vi "例4-20.vi"   [LabVIEW 2019]
uses:
  <vilib>/Utility/file.llb/Write Delimited Spreadsheet (DBL).vi
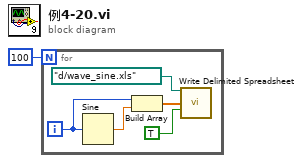
[diagram p0: block diagram]
diagram:
  n1 = for {
    N: 100 -> [_]
    i -> [w2]
    n2 = Sine(x=w2) -> (sin(x)=w5:dbl)
    n3 = Build Array(w2, w5) -> (w4:dbl[])
    n4 = call-poly <vilib>:"Write Delimited Spreadsheet.vi"("file path (dialog if empty)"=path "d:/wave_sine.xls", "1D data"=w4, "append to file? (new file:F)"=TRUE) -> ()  [unwired: 11 in, 2 out]
  }
